vi "Obtain JKISM Message Event.vi"(8 "error in (no error)":errorcluster, 11 "Module":string) -> (0 "error out":errorcluster, 3 "JKISM Message Event":refnum<user-event>)   [LabVIEW 2017, in "JKISM Message Event.lvlib"]
uses:
  JKISM Message Event.lvlib
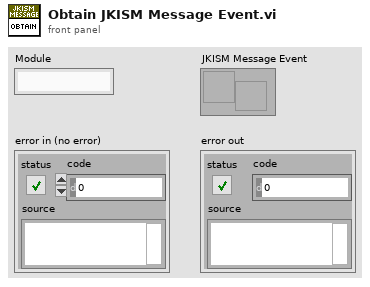
[diagram p1: front panel]
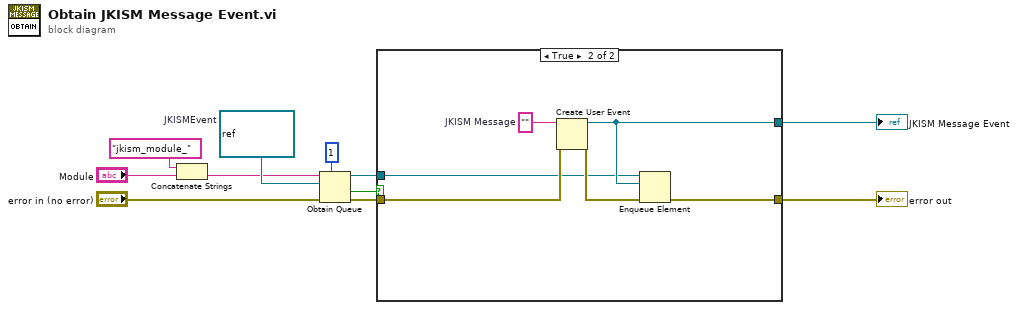
[diagram p0: block diagram]
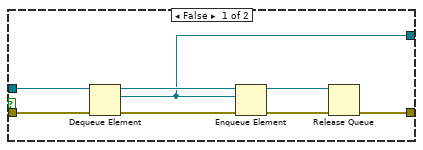
[diagram p2: hidden frame]
diagram:
  w5 = refnum<user-event> refnum  # JKISMEvent
  n1 = Concatenate Strings("jkism_module_" ("string"), "Module") -> (w3:string)
  n2 = Obtain Queue(max queue size (-1, unlimited)=1, name (unnamed)=w3, element data type=w5, error in (no error)="error in (no error)") -> (queue out=w7:refnum<queue>, created new?=w4:bool, error out=w9:errorcluster)  [unwired: 1 in]
  n3 = case shown="True" w4 {
    tunnel: [w12 w25] -> w1
    tunnel: w9 -> [w19 w23]
    tunnel: [w15 w22] -> w8
    tunnel: w7 -> [w17 w21]
    frame False {
      n4 = Dequeue Element(queue=w17, error in (no error)=w19) -> (queue out=w16:refnum<queue>, element=w15:refnum<user-event>, error out=w18:errorcluster)  [unwired: 1 in, 1 out]
      n5 = Enqueue Element(queue=w16, element=w15, error in (no error)=w18) -> (queue out=w14:refnum<queue>, error out=w13:errorcluster)  [unwired: 1 in, 1 out]
      n6 = Release Queue(queue=w14, error in (no error)=w13) -> (error out=w12:errorcluster)  [unwired: 1 in, 2 out]
    }
    frame True {
      w20 = ""  # JKISM Message
      n7 = Create User Event(user event datatype=w20, error in=w23) -> (user event=w22:refnum<user-event>, error out=w24:errorcluster)
      n8 = Enqueue Element(queue=w21, element=w22, error in (no error)=w24) -> (error out=w25:errorcluster)  [unwired: 1 in, 2 out]
    }
  }
  "error out" <- w1
  "JKISM Message Event" <- w8
